vi "ReadSerial.vi"(8 "error in":errorcluster) -> ()   [LabVIEW 2015]
uses:
  Sensor data.ctl
  <vilib>/Rock Robotics/SystemInterfaces/i2clib/i2c_bus.ctl
panel:
  out "Encoder":T1
  out "Switch":T1
  out "Last Sensor Data Received":T1
  out "Sequence":dbl
  out "Status":dbl
  out "Has Connection":bool
  out "Message Data":u8[](array[numeric])
  out "Message Length":u8
  out "Message Type":u8
  in  "Reset":bool
  out "error out":errorcluster
  out "output array":u8[](array[numeric])
  # "Keep Alive Packet"
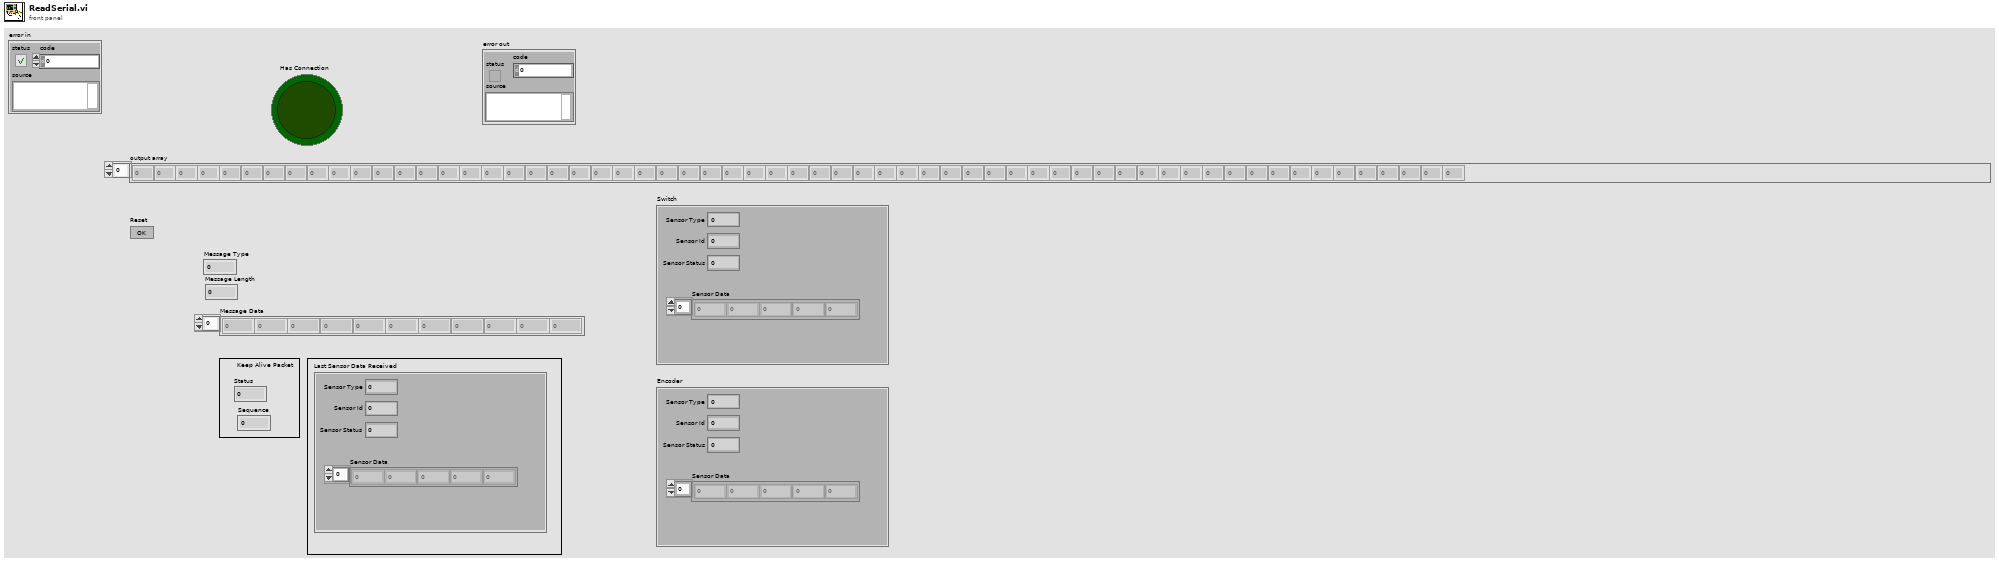
[diagram p1: front panel]
types:
  T1 = typedef "Sensor data.ctl" = cluster{"Sensor Type":dbl, "Sensor Id":dbl, "Sensor Status":dbl, "Sensor Data":u8[]}
  T2 = typedef "i2c_bus.ctl" = enum16{"I2C On-Board", "I2C MXP", "Invalid"}
  T3 = typedef "WPI_I2CDevRef.ctl" = cluster{"DevStatus":errorcluster, "Device Address":u8, "Handle":i32, "I2C Bus":T2}
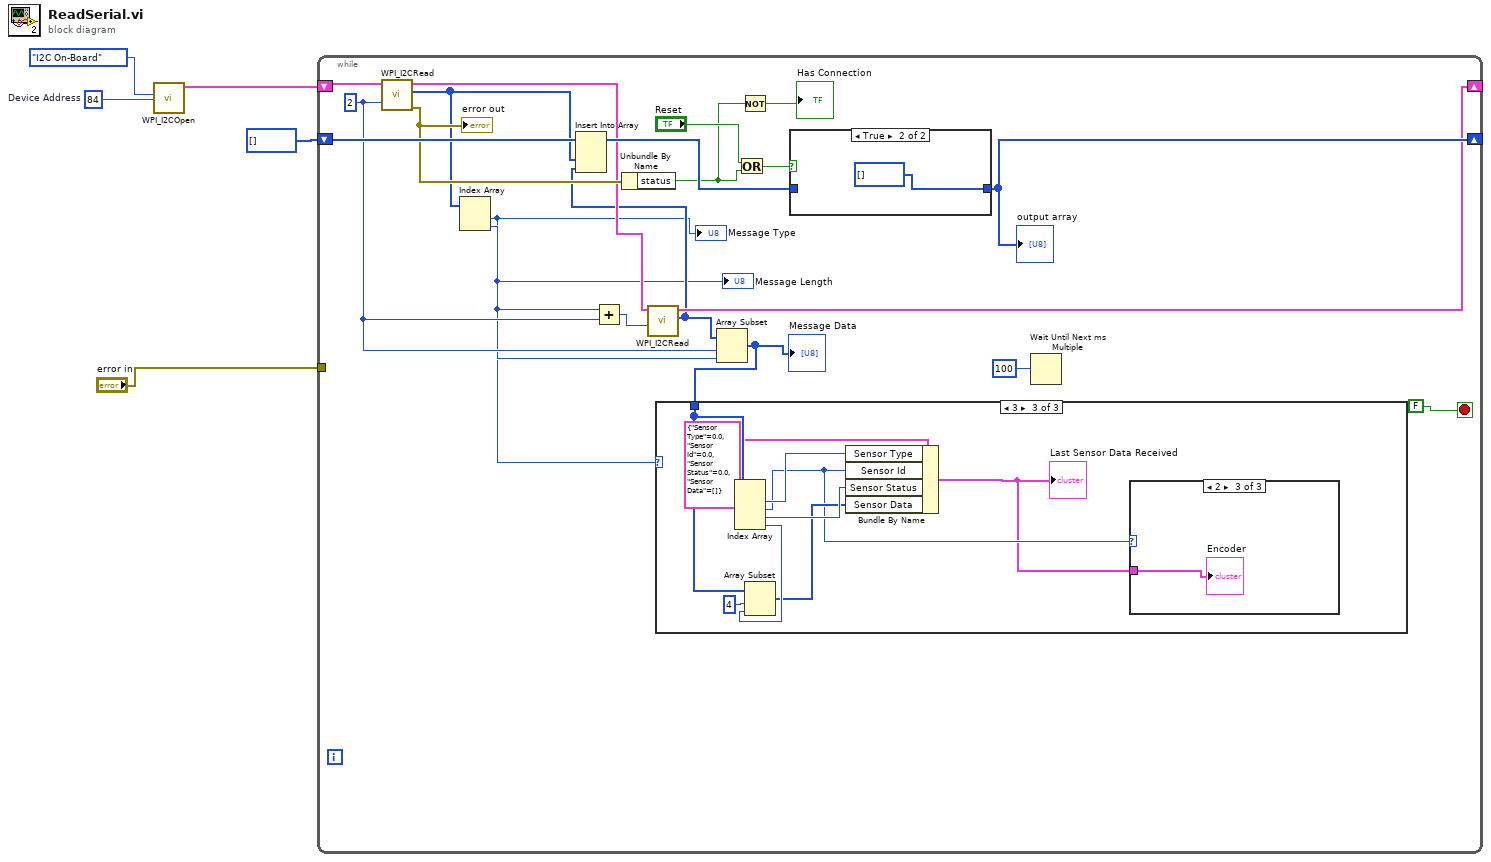
[diagram p0: block diagram]
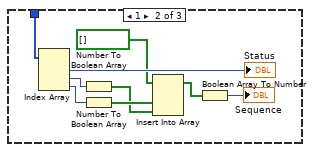
[diagram p3: hidden frame]
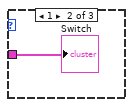
[diagram p5: hidden frame]
diagram:
  w2 = u8 84  # Device Address
  n1 = call <vilib>:"WPI_I2COpen.vi"("Device Address"=w2, "I2C Bus"=i2c_bus."I2C On-Board") -> ("I2CDevRef"=w4:T3)  [unwired: 8 in, 1 out]
  n2 = while {
    shift-right: [w20] -> _
    shift-left: u8[] [] ("byte array 2") -> [w24]
    shift-right: [w14] -> _
    shift-left: w4 -> [w23]
    tunnel: "error in" -> [_]
    stop <- FALSE stop-if-true
    w11 = u8 2 ("I2CBytesToRead")
    n3 = call <vilib>:"WPI_I2CRead.vi"("I2CBytesToRead"=w11, "I2CDevRef"=w23) -> ("error out"=w19:errorcluster, "Data Out"=w16:u8[], "I2CDevRef"=w15:T3)  [unwired: 7 in]
    "error out" <- w19
    n4 = Index Array(array=w16) -> (element #1=w7:u8, element #2=w10:u8)  [unwired: 2 in]
    "Message Type" <- w7
    "Message Length" <- w10
    n5 = Add(x=w10, y=w11) -> (x+y=w13:u8)
    n6 = Unbundle By Name(w19) -> ("status"=w8:bool)
    n7 = call <vilib>:"WPI_I2CRead.vi"("I2CBytesToRead"=w13, "I2CDevRef"=w15) -> ("Data Out"=w12:u8[], "I2CDevRef"=w14:T3)  [unwired: 7 in, 1 out]
    n8 = Insert Into Array(array=w24, new element #1=w16, new element #2=w12) -> (w21:u8[])  [unwired: 1 in]
    n9 = Array Subset(array=w12, index=w11, length=w10) -> (w6:u8[])
    "Message Data" <- w6
    n10 = case shown="3" w7 {
      tunnel: w6 -> [_ w33 w43]
      frame 0, Default {
      }
      frame 1 {
        n11 = Index Array(array=w33) -> (element #1=→"Status":u8, element #2=w31:u8, element #3=w30:u8)  [unwired: 3 in]
        n12 = Number To Boolean Array(number=w31) -> (Boolean array=w26:bool[])
        n13 = Number To Boolean Array(number=w30) -> (Boolean array=w27:bool[])
        n14 = Insert Into Array(array=bool[] [] ("Boolean array"), new element #1=w27, new element #2=w26) -> (w28:bool[])  [unwired: 1 in]
        n15 = Boolean Array To Number(Boolean array=w28) -> (number=→"Sequence":u32)
      }
      frame 3 {
        n16 = Index Array(array=w43) -> (element #1=w38:u8, element #2=w36:u8, element #3=w39:u8, element #4=w41:u8)  [unwired: 4 in]
        n17 = Array Subset(array=w43, index=4, length=w41) -> (w37:u8[])
        n18 = Bundle By Name(cluster=T1 {"Sensor Type"=0.0, "Sensor Id"=0.0, "Sensor Status"=0.0, "Sensor Data"=[]} ("Sensor Data"), "Sensor Type"=w38, "Sensor Id"=w36, "Sensor Status"=w39, "Sensor Data"=w37) -> (w35:T1)
        "Last Sensor Data Received" <- w35
        n19 = case shown="2" w36 {
          tunnel: w35 -> [_ w44 w45]
          frame 0, Default {
          }
          frame 1 {
            "Switch" <- w44
          }
          frame 2 {
            "Encoder" <- w45
          }
        }
      }
    }
    n20 = Or(x="Reset", y=w8) -> (x .or. y?=w17:bool)
    n21 = Not(x=w8) -> (.not. x?=→"Has Connection":bool)
    n22 = case shown="True" w17 {
      tunnel: w21 -> [w46 _]
      tunnel: [w46 u8[] [] ("byte array 2")] -> w20
      frame False {
      }
      frame True {
      }
    }
    "output array" <- w20
    n23 = Wait Until Next ms Multiple(millisecond multiple=100) -> ()  [unwired: 1 out]
  }
